vi "sandbox.vi"() -> ()   [LabVIEW 2019, in "SharedVariableWrapper.lvclass"]
uses:
  SharedVariableWrapper.lvclass
  Logger_class/Current Alarms.ctl
  Logger_class/EventData.ctl
  TypeDef/AlarmType.ctl
  SharedVariableWrapper.lvclass/SharedVariableWrapper.ctl
  78131cf0-57b9-4322-b737-fe0b31e0abb3.vi
  d8354c83-9461-4e26-96e5-08e4d70f2563.vi
  d8354c83-9461-4e26-96e5-08e4d70f2563.vi/9f709bea-a1f0-4727-aaf6-6718a334b044.vi
  Write Var Info.vi
  Read Var Info.vi
  Read connection str.vi
  <userlib>/_OpenG.lib/time/time.llb/Tick Count (ms)__ogtk.vi
panel:
  in  "Multicolumn Listbox":i32(listbox)=-1
  out "data out":T1
  in  "stop":bool
  out "connected":bool
  out "dt read":u32
  out "error out 2":errorcluster
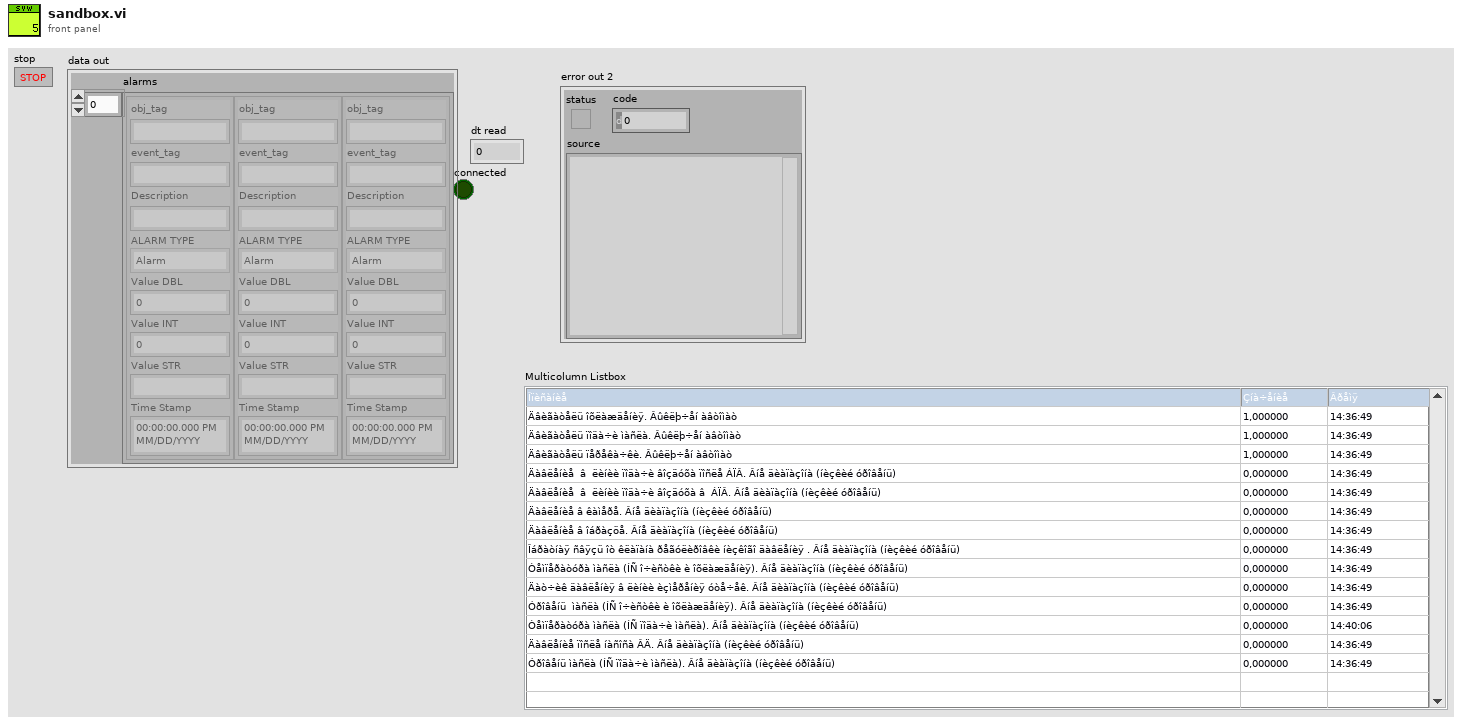
[diagram p1: front panel]
types:
  T1 = typedef "Current Alarms.ctl" = cluster{"alarms":T2[]}
  T2 = typedef "EventData.ctl" = cluster{"obj_tag":string, "event_tag":string, "Description":string, "ALARM TYPE":T3, "Value DBL":dbl, "Value INT":i32, "Value STR":string, "Time Stamp":timestamp}
  T3 = typedef "AlarmType.ctl" = enum16{"Normal", "Warning", "Alarm"}
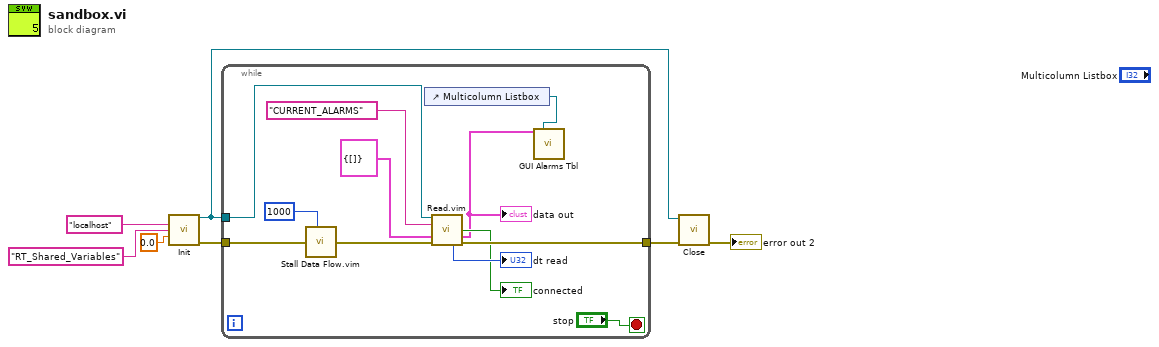
[diagram p0: block diagram]
diagram:
  n1 = call "Init.vi"("host"="localhost", "lib"="RT_Shared_Variables", "update timeout"=0.0) -> ("SVW"=w1:refnum<class "SharedVariableWrapper.lvclass">, "error out"=w3:errorcluster)  [unwired: 11 in]
  n2 = while {
    tunnel: [w17] -> w5
    tunnel: w3 -> [w14]
    tunnel: w1 -> [w13]
    stop <- "stop" stop-if-true
    n3 = call "Stall Data Flow.vim"("value in"=w14, "milliseconds to wait"=u32 1000) -> ("value out"=w12:errorcluster)  [unwired: 1 out]
    n4 = control-ref of="Multicolumn Listbox"() -> (w8:refnum<vi>)
    n5 = call "Read.vim"("SharedVariableWrapper in"=w13, "name"="CURRENT_ALARMS", "DataType"=T1 {"alarms"=[]} ("Current Alarms"), "error in (no error)"=w12) -> ("connected"=→"connected":bool, "data out"=w9:T1, "dt read"=→"dt read":u32, "error out"=w17:errorcluster)  [unwired: 5 in, 3 out]
    "data out" <- w9
    n6 = call "GUI Alarms Tbl.vi"("data in"=w9, "Multicolumn Listbox ref"=w8) -> ()  [unwired: 14 in]
  }
  n7 = call "Close.vi"("error in (no error)"=w5, "SharedVariableWrapper in"=w1) -> ("error out"=→"error out 2":errorcluster)  [unwired: 8 in, 1 out]
